vi "waitNotifierStopServer.vi"(8 "error in (no error)":errorcluster, 11 "TcpServerTel in":refnum<class "TcpServerTel.lvclass">) -> (0 "error out":errorcluster, 2 "stopServer":bool, 3 "TcpServerTel out":refnum<class "TcpServerTel.lvclass">)   [LabVIEW 2018, in "TcpServerTel.lvclass"]
doc: "Wait to stop the runServer.vi. This is a non-block call function."
uses:
  TcpServerTel.lvclass
  home/pcortes/Documents/github/ts_labview_tcp_json/src/TcpServerBase/TcpServerBase.lvclass
  TcpServerBase/TcpServerBase.lvclass/TcpServerBase.ctl
  TcpServerBase/TcpServerBase.lvclass
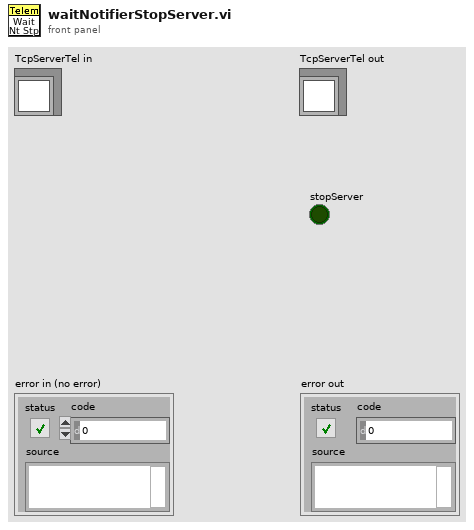
[diagram p1: front panel]
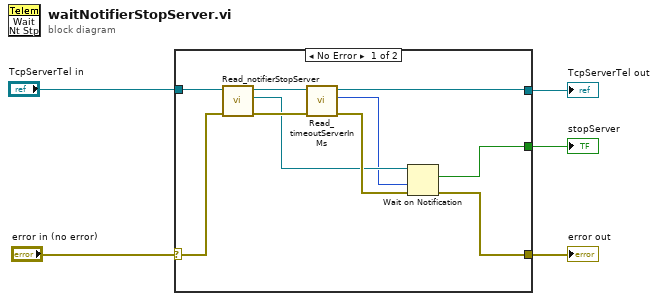
[diagram p0: block diagram]
diagram:
  n1 = case shown="No Error" "error in (no error)" {
    selector: "error in (no error)" -> [w10 w17]
    tunnel: "TcpServerTel in" -> [w11 w16]
    tunnel: [w15 w17] -> w3
    tunnel: [w9 w16] -> w2
    tunnel: [w14 _] -> w1
    frame No Error {
      n2 = call "Read_notifierStopServer.vi"("error in (no error)"=w10, "TcpServerBase in"=w11) -> ("error out"=w12:errorcluster, "notifierStopServer"=w7:refnum<notifier>, "TcpServerBase out"=w13:refnum<class "TcpServerTel.lvclass">)  [unwired: 7 in]
      n3 = call "Read_timeoutServerInMs.vi"("error in (no error)"=w12, "TcpServerBase in"=w13) -> ("error out"=w8:errorcluster, "timeoutServerInMs"=w6:i32, "TcpServerBase out"=w9:refnum<class "TcpServerTel.lvclass">)  [unwired: 7 in]
      n4 = Wait on Notification(notifier=w7, timeout in ms (-1)=w6, error in (no error)=w8) -> (notification=w14:bool, error out=w15:errorcluster)  [unwired: 1 in, 2 out]
    }
    frame Error {
    }
  }
  "error out" <- w3
  "TcpServerTel out" <- w2
  "stopServer" <- w1
